vi "SetEnumFeatureSymbol.vi"(8 "pEnumSymbol":string, 9 "pFeatureName":string, 10 "handle":i64, 11 "error in (no error)":errorcluster) -> (2 "return type":i32, 3 "error out":errorcluster)   [LabVIEW 2016]
uses:
  MVSDKmd.dll
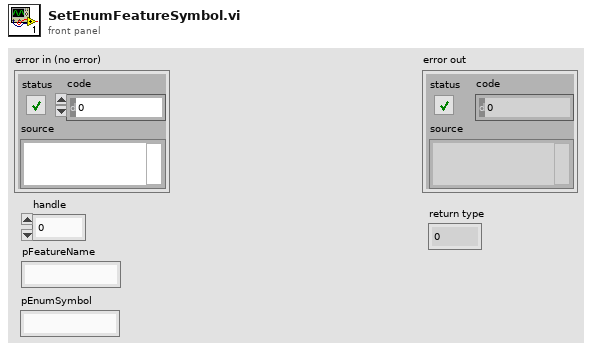
[diagram p1: front panel]
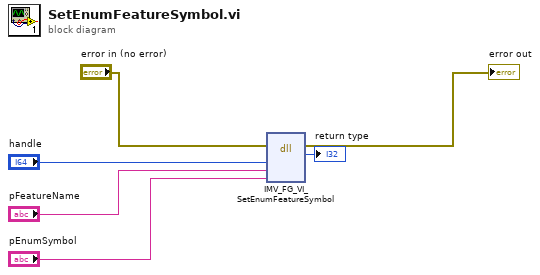
[diagram p0: block diagram]
diagram:
  n1 = dll-call lib="MVSDKmd.dll" fn="IMV_FG_VI_SetEnumFeatureSymbol"(error in="error in (no error)", "handle"="handle", "pFeatureName"="pFeatureName", "pEnumSymbol"="pEnumSymbol") -> (error out=→"error out":errorcluster, "return type"=→"return type":i32)  [unwired: 5 in, 1 out]
